vi "ApplyPict.vi"(8 "error in (no error)":errorcluster, 11 "Sudoku in":refnum<class "Sudoku.lvclass">) -> (0 "error out":errorcluster, 3 "Sudoku out":refnum<class "Sudoku.lvclass">)   [LabVIEW 2021, in "Sudoku.lvclass"]
uses:
  Sudoku.lvclass
  Sudoku.lvclass/Sudoku.ctl
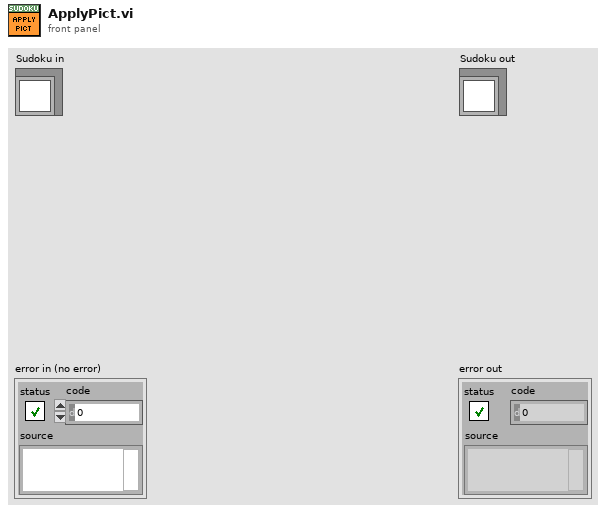
[diagram p1: front panel]
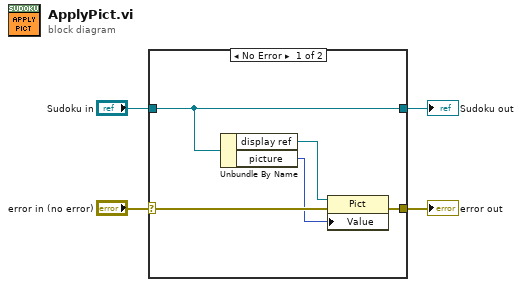
[diagram p0: block diagram]
diagram:
  n1 = case shown="No Error" "error in (no error)" {
    selector: "error in (no error)" -> [w7 w11]
    tunnel: [w5 w11] -> w3
    tunnel: [w9 w10] -> w1
    tunnel: "Sudoku in" -> [w9 w10]
    frame No Error {
      n2 = Unbundle By Name(w9) -> ("display ref"=w8:refnum<vi>, "picture"=w6:picture)
      n3 = property class="Pict"(reference=w8, error in=w7, "Value"=w6) -> (error out=w5:errorcluster)  [unwired: 1 out]
    }
    frame Error {
    }
  }
  "error out" <- w3
  "Sudoku out" <- w1
